vi "PE Get System Name.vi"(8 "error in (no error)":errorcluster, 10 "index":i32, 11 "peHandle":u32) -> (0 "error out":errorcluster, 2 "peHandle 2":u32, 3 "name":string)   [LabVIEW 2017, in "PE_Filter_SDK.lvlib"]
doc: "PEFILTERSDK_API PE_STATUS PE_GetSystemName(CPE_HANDLE peHandle, int index, char* name, int size);"
uses:
  PE_Filter_SDK.lvlib
  PE_Filter_SDK.dll
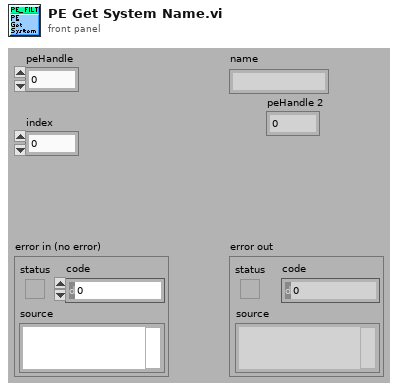
[diagram p1: front panel]
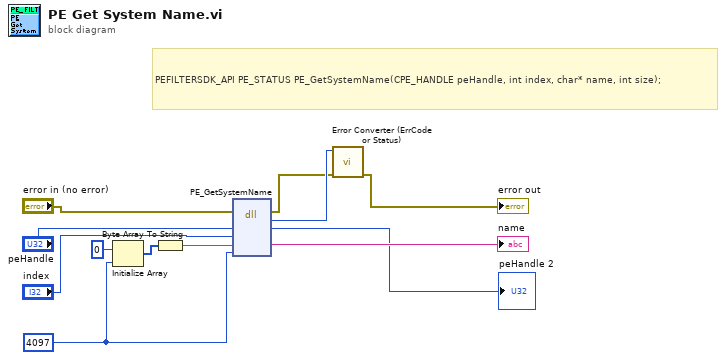
[diagram p0: block diagram]
diagram:
  w8 = 4097 ("size")
  # "PEFILTERSDK_API PE_STATUS PE_GetSystemName(CPE_HANDLE peHandle, int index, char* name, int size);"
  n1 = Initialize Array(u8 0 ("element"), w8) -> (w10:u8[])
  n2 = Byte Array To String(unsigned byte array=w10) -> (string=w9:string)
  n3 = dll-call lib="PE_Filter_SDK.dll" fn="PE_GetSystemName"(error in="error in (no error)", "peHandle"="peHandle", "index"="index", "name"=w9, "size"=w8) -> (error out=w3:errorcluster, "return type"=w4:u32, "peHandle"=→"peHandle 2":u32, "name"=→"name":string)  [unwired: 4 in, 1 out]
  n4 = call "Error Converter (ErrCode or Status).vi"("error in (no error)"=w3, "error code"=w4) -> ("error out"=→"error out":errorcluster)  [unwired: 9 in]
